vi "Prepare_For_Consolidated_Save.vi"(7 "inside target file":bool, 8 "error in (no error)":errorcluster, 11 "AB_Source_Library in":refnum<class "AB_Source_Library.lvclass">) -> (0 "error out":errorcluster, 2 "item_Data":T1, 3 "AB_Source_Library out":refnum<class "AB_Source_Library.lvclass">)   [LabVIEW 2020, in "AB_Source_Library.lvclass"]
uses:
  <vilib>/AppBuilder/AB_Classes/Source/Library/AB_Source_Library.lvclass
  <vilib>/AppBuilder/Engine/AB_Engine_Consolidated_Save_Item_Info.ctl
  <vilib>/AppBuilder/AB_Classes/Source/Library/AB_Source_Library.lvclass/AB_Source_Library.ctl
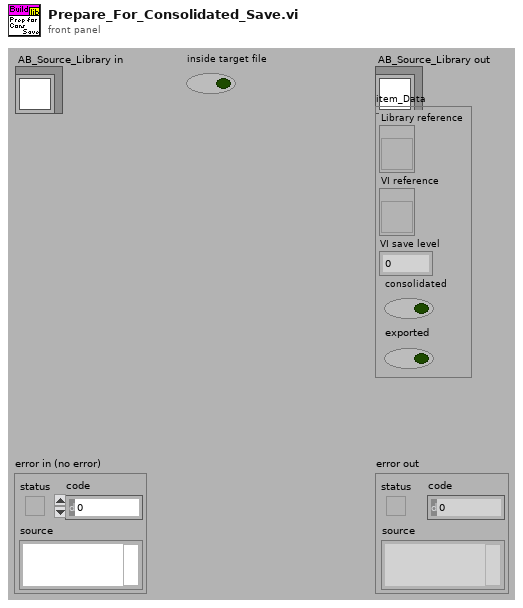
[diagram p1: front panel]
types:
  T1 = typedef "AB_Engine_Consolidated_Save_Item_Info.ctl" = cluster{"Library reference":refnum<vi>, "VI reference":refnum<vi>, "VI save level":i32, "consolidated":bool, "exported":bool}
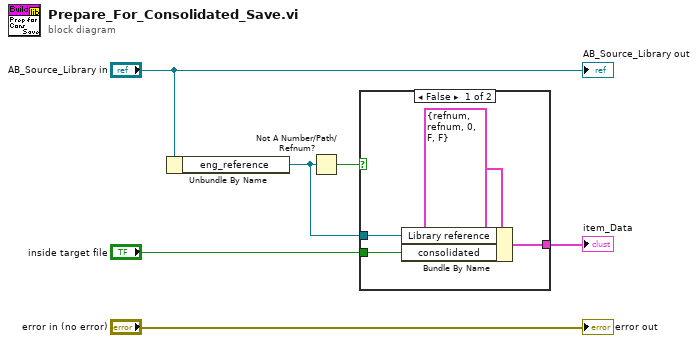
[diagram p0: block diagram]
diagram:
  n1 = Unbundle By Name("AB_Source_Library in") -> ("eng_reference"=w3:refnum<vi>)
  n2 = Not A Number/Path/Refnum?(number/path/refnum=w3) -> (NaN/Path/Refnum?=w4:bool)
  n3 = case shown="False" w4 {
    tunnel: w3 -> [w9 _]
    tunnel: [w8 _] -> w2
    tunnel: "inside target file" -> [w7 _]
    frame False {
      n4 = Bundle By Name(cluster=T1 {"Library reference"=refnum, "VI reference"=refnum, "VI save level"=0, "consolidated"=FALSE, "exported"=FALSE} ("item_Data"), "Library reference"=w9, "consolidated"=w7) -> (w8:T1)
    }
    frame True {
    }
  }
  "item_Data" <- w2
  "error out" <- "error in (no error)"
  "AB_Source_Library out" <- "AB_Source_Library in"
